vi "A_5.vi"() -> ()   [LabVIEW 2020]
uses:
  <vilib>/Analysis/NI_AALBase.lvlib
panel:
  in  "Loop delay [ms]":u32
  in  "stop":bool
  in  "Duty cycle [%]":dbl
  out "Waveform Chart":dbl[](graph)
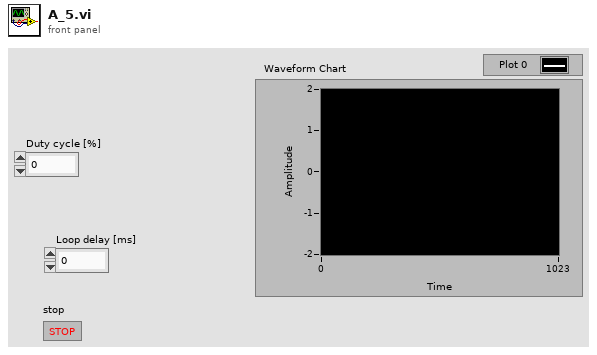
[diagram p1: front panel]
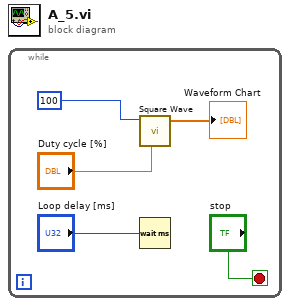
[diagram p0: block diagram]
diagram:
  n1 = while {
    stop <- "stop" stop-if-true
    n2 = call <vilib>:"Square Wave.vi"("samples"=100, "duty cycle (%)"="Duty cycle [%]") -> ("square wave"=→"Waveform Chart":dbl[])  [unwired: 4 in, 2 out]
    n3 = Wait (ms)(milliseconds to wait="Loop delay [ms]") -> ()  [unwired: 1 out]
  }
